vi "oa_TV Decimate N (1Chan).vi"(5 "reset? (F)":bool, 8 "error in (no error)":errorcluster, 10 "pulse/revolution":i32, 11 "pulse positions [s]":dbl[](array[numeric])) -> (0 "error out":errorcluster, 1 "revolution index":i32, 2 "revolution":i32, 3 "pulse positions":dbl[](array[numeric]))   [LabVIEW 2017, in "SoundVib_Torsional.lvlib"]
uses:
  <vilib>/addons/Sound and Vibration/Order Analysis/Torsional Vibration/SoundVib_Torsional.lvlib
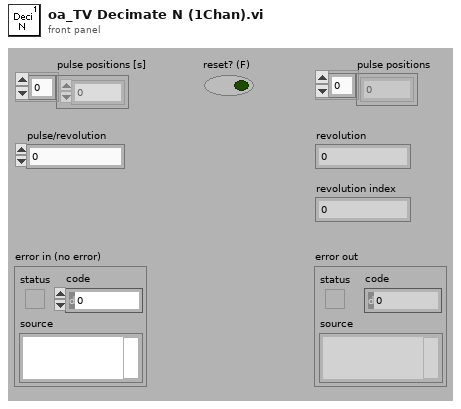
[diagram p1: front panel]
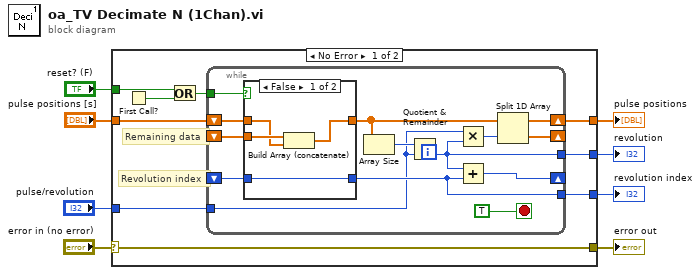
[diagram p0: block diagram]
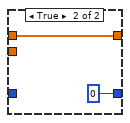
[diagram p2: hidden frame]
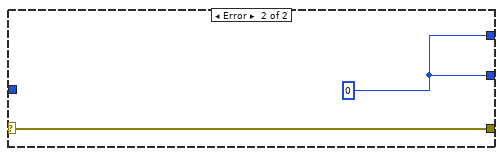
[diagram p3: hidden frame]
diagram:
  n1 = case shown="No Error" "error in (no error)" {
    selector: "error in (no error)" -> [w17 w39]
    tunnel: [w17 w39] -> w7
    tunnel: "pulse positions [s]" -> [w15 _]
    tunnel: "pulse/revolution" -> [w16 _]
    tunnel: [w11 _] -> w4
    tunnel: [w14 w38] -> w3
    tunnel: [w10 w38] -> w2
    tunnel: "reset? (F)" -> [w9 _]
    frame No Error {
      # "Revolution index"
      # "Remaining data"
      n2 = First Call?() -> (First Call?: T/F=w13:bool)
      n3 = Or(x=w9, y=w13) -> (x .or. y?=w12:bool)
      n4 = while {
        tunnel: w16 -> [w20]
        tunnel: [w24] -> w14
        tunnel: w12 -> [w29]
        shift-right: [w21] -> _
        shift-left: _ -> [w27]
        shift-right: [w26] -> _
        shift-left: _ -> [w25]
        tunnel: [w18] -> w10
        shift-right: [w19] -> w11
        shift-left: w15 -> [w28]
        stop <- TRUE stop-if-true
        n5 = case shown="False" w29 {
          tunnel: [w33 w37] -> w22
          tunnel: w28 -> [w34 w37]
          tunnel: w27 -> [w35 _]
          tunnel: w25 -> [w32 _]
          tunnel: [w32 0] -> w24
          frame False {
            n6 = Build Array (concatenate)(w35, w34) -> (w33:dbl[])
          }
          frame True {
          }
        }
        n7 = Array Size(array=w22) -> (size(s)=w31:i32)
        n8 = Quotient & Remainder(x=w31, y=w20) -> (floor(x/y)=w18:i32)  [unwired: 1 out]
        n9 = Multiply(x=w20, y=w18) -> (x*y=w23:i32)
        n10 = Add(x=w18, y=w24) -> (x+y=w26:i32)
        n11 = Split 1D Array(array=w22, index=w23) -> (first subarray=w19:dbl[], second subarray=w21:dbl[])
      }
    }
    frame Error {
      w38 = 0
    }
  }
  "error out" <- w7
  "pulse positions" <- w4
  "revolution index" <- w3
  "revolution" <- w2
